vi "To Generic.vi"(8 "error in (no error)":errorcluster, 11 "Request Data in":refnum<class "Timed Data.lvclass">) -> (0 "error out":errorcluster, 2 "Generic Data":refnum<class "Generic Data.lvclass">[](array[class]), 3 "Data Name":string[](array[string]))   [LabVIEW 2020, in "Publisher.lvlib" / "Timed Data.lvclass"]
doc: "Present private data as an array of named generic data elements."
uses:
  Timed Data.lvclass
  PPL/HDH.Data.Generic.lvlibp/Generic Data/Generic Data.lvclass
  Timed Data.lvclass/Timed Data.ctl
  PPL/HDH.Data.Generic.lvlibp/Generic Data/Time Stamp/Time Stamp.lvclass
  C:/Current projects/WS/PPL/HDH.Data.Generic.lvlibp/Generic Data/Generic Data.lvclass
  PPL/HDH.Data.Generic.lvlibp/Generic Data/U32/U32.lvclass
  PPL/HDH.Data.Generic.lvlibp/Generic Data/Double/Double.lvclass
  PPL/HDH.Data.Generic.lvlibp/Data.lvclass
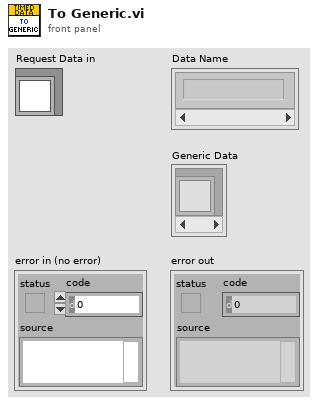
[diagram p1: front panel]
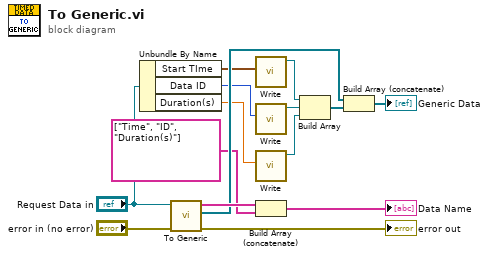
[diagram p0: block diagram]
diagram:
  n1 = Unbundle By Name("Request Data in") -> ("Start TIme"=w11:timestamp, "Data ID"=w9:u32, "Duration(s)"=w7:dbl)
  n2 = call-parent "To Generic.vi"("error in (no error)"="error in (no error)", "Data in"="Request Data in") -> ("error out"=→"error out":errorcluster, "Generic Data"=w14:refnum<class "Generic Data.lvclass">[], "Data Name"=w15:string[])  [unwired: 7 in]
  n3 = call "Write.vi"("Time Stamp"=w11) -> ("Time Stamp out"=w10:refnum<class "Time Stamp.lvclass">)  [unwired: 10 in]
  n4 = call "Write.vi"("U32"=w9) -> ("U32 out"=w8:refnum<class "U32.lvclass">)  [unwired: 10 in]
  n5 = call "Write.vi"("Double"=w7) -> ("Double out"=w6:refnum<class "Double.lvclass">)  [unwired: 10 in]
  n6 = Build Array (concatenate)(w15, string[] ["Time", "ID", "Duration(s)"] ("array")) -> (→"Data Name":string[])
  n7 = Build Array(w10, w8, w6) -> (w5:refnum<class "Generic Data.lvclass">[])
  n8 = Build Array (concatenate)(w14, w5) -> (→"Generic Data":refnum<class "Generic Data.lvclass">[])
